vi "Global - All UI Loop Stop.vi"() -> ()   [LabVIEW 2015]
panel:
  out "Connection Status":bool caption="连接状态"
  in  "All UI Loop Stop":bool caption="全部UI循环停止"
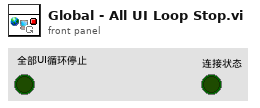
[diagram p1: front panel]
diagram:
